vi "Run and Open from Async Call.vi"(7 "UI Top Ref":refnum<vi>, 8 "error in (no error)":errorcluster, 11 "Async Call Ref":refnum<vi>) -> (0 "error out":errorcluster)   [LabVIEW 2024, in "User Interface.lvlib"]
uses:
  User Interface.lvlib
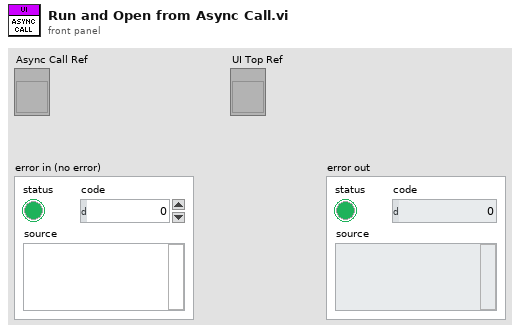
[diagram p1: front panel]
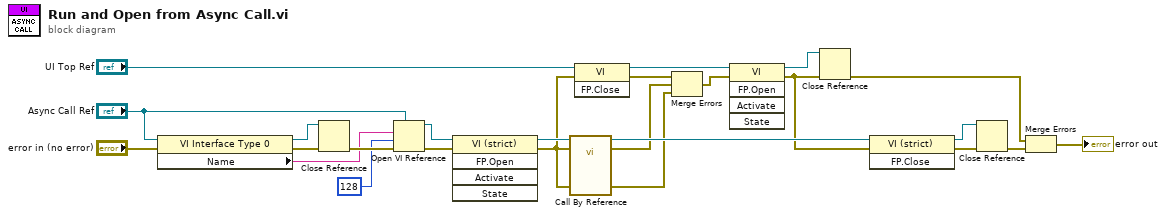
[diagram p0: block diagram]
diagram:
  n1 = property class="VI Interface Type 0"(reference="Async Call Ref", error in="error in (no error)") -> (reference out=w23:refnum<vi>, error out=w24:errorcluster, "Name"=w22:string)
  n2 = Close Reference(reference=w23, error in (no error)=w24) -> (error out=w25:errorcluster)
  n3 = Open VI Reference(type specifier VI Refnum (for type only)="Async Call Ref", vi path=w22, options=128, error in (no error)=w25) -> (vi reference=w20:refnum<vi>, error out=w21:errorcluster)  [unwired: 2 in]
  n4 = invoke class="VI (strict)" method="FP.Open"(reference=w20, error in=w21) -> (reference out=w19:refnum<vi>, error out=w9:errorcluster)  [unwired: 3 in, 3 out]
  n5 = call-by-ref "?"(reference=w19, error in=w9, "error in"=w9) -> (reference out=w16:refnum<vi>, error out=w7:errorcluster, 0:"error out"=w6:errorcluster)  [unwired: 10 in]
  n6 = invoke class="VI" method="FP.Close"(reference="UI Top Ref", error in=w9) -> (reference out=w10:refnum<vi>, error out=w8:errorcluster)  [unwired: 1 in, 1 out]
  n7 = Merge Errors(w8, w7, w6) -> (w5:errorcluster)
  n8 = invoke class="VI" method="FP.Open"(reference=w10, error in=w5) -> (reference out=w13:refnum<vi>, error out=w4:errorcluster)  [unwired: 3 in, 3 out]
  n9 = Close Reference(reference=w13, error in (no error)=w4) -> (error out=w3:errorcluster)
  n10 = invoke class="VI (strict)" method="FP.Close"(reference=w16, error in=w4) -> (reference out=w15:refnum<vi>, error out=w1:errorcluster)  [unwired: 1 in, 1 out]
  n11 = Close Reference(reference=w15, error in (no error)=w1) -> (error out=w18:errorcluster)
  n12 = Merge Errors(w3, w18) -> (→"error out":errorcluster)
